vi "Sub_Accelerometer.vi"(11 "Refnum in":refnum<k21>) -> (0 "error out":errorcluster, 2 "data":dbl[](array[numeric]), 3 "Refnum out":refnum<k21>)   [LabVIEW 2014]
uses:
  <vilib>/DAQmx/read.llb/DAQmx Read (Analog 1D DBL 1Chan NSamp).vi
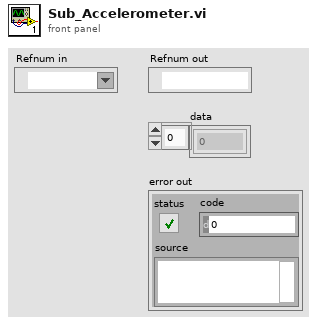
[diagram p1: front panel]
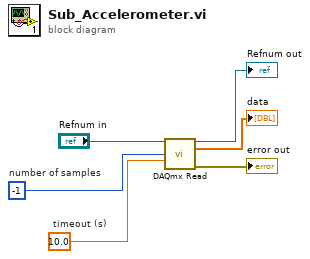
[diagram p0: block diagram]
diagram:
  w2 = 10.0  # timeout (s)
  w1 = -1  # number of samples
  n1 = call-poly <vilib>:"DAQmx Read.vi"("task/channels in"="Refnum in", "number of samples per channel"=w1, "timeout"=w2) -> ("task out"=→"Refnum out":refnum<k21>, "data"=→"data":dbl[], "error out"=→"error out":errorcluster)  [unwired: 10 in]
